vi "tra25cc_goto_xy-relative.vi"(8 "error in (no error)":errorcluster, 10 "xy_val":cluster{"x_val":dbl, "y_val":dbl}, 11 "conn_xyz_in":T2) -> (0 "error out":errorcluster, 3 "conn_xyz_out":T1)   [LabVIEW 2014]
uses:
  D:/Microscope/Software/Tools/Stage_xyz/Dll/Newport.CONEXCC.CommandInterface.dll
  Dll/Newport.CONEXCC.CommandInterface.dll
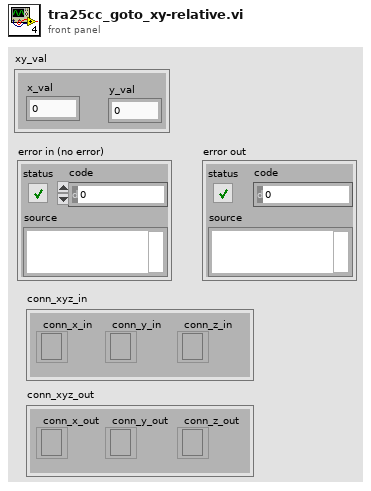
[diagram p1: front panel]
types:
  T1 = cluster{"conn_x_out":refnum<k24>, "conn_y_out":refnum<k24>, "conn_z_out":refnum<k24>}
  T2 = cluster{"conn_x_in":refnum<k24>, "conn_y_in":refnum<k24>, "conn_z_in":refnum<k24>}
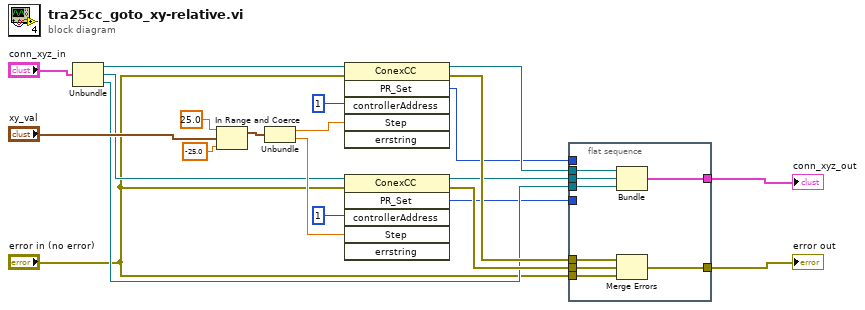
[diagram p0: block diagram]
diagram:
  n1 = Unbundle("conn_xyz_in") -> ("conn_x_in"=w8:refnum<k24>, "conn_y_in"=w7:refnum<k24>, "conn_z_in"=w6:refnum<k24>)
  n2 = In Range and Coerce(upper limit=25.0, x="xy_val", lower limit=-25.0) -> (coerced(x)=w11:cluster{"x_val":dbl, "y_val":dbl})  [unwired: 1 out]
  n3 = Unbundle(w11) -> ("x_val"=w16:dbl, "y_val"=w15:dbl)
  n4 = invoke class="ConexCC" method="PR_Set"(reference=w8, error in="error in (no error)", "controllerAddress"=1, "Step"=w16) -> (reference out=w14:refnum<k24>, error out=w18:errorcluster, "PR_Set"=w2:i32)  [unwired: 2 in, 3 out]
  n5 = invoke class="ConexCC" method="PR_Set"(reference=w7, error in="error in (no error)", "controllerAddress"=1, "Step"=w15) -> (reference out=w13:refnum<k24>, error out=w19:errorcluster, "PR_Set"=w1:i32)  [unwired: 2 in, 3 out]
  n6 = flat-sequence {
    tunnel: w19 -> [w29]
    tunnel: w18 -> [w28]
    tunnel: w14 -> [w27]
    tunnel: w13 -> [w26]
    tunnel: w6 -> [w25]
    tunnel: "error in (no error)" -> [w24]
    tunnel: [w23] -> w4
    tunnel: [w22] -> w3
    tunnel: w2 -> [_]
    tunnel: w1 -> [_]
    frame #0 {
      n7 = Bundle("conn_x_in"=w27, "conn_y_in"=w26, "conn_z_in"=w25) -> (w23:T2)  [unwired: 1 in]
      n8 = Merge Errors(w28, w29, w24) -> (w22:errorcluster)
    }
  }
  "error out" <- w3
  "conn_xyz_out" <- w4
